vi "Add(U8).vi"(1 "Enable(T)":bool=TRUE, 2 "In":u8, 4 "n":u8=1) -> (6 "Out":u8=1)   [LabVIEW 2013]
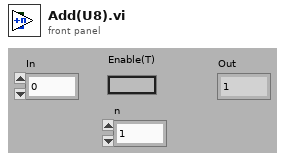
[diagram p1: front panel]
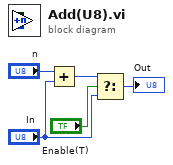
[diagram p0: block diagram]
diagram:
  n1 = Add(x="n", y="In") -> (x+y=w1:u8)
  n2 = Select(t=w1, s="Enable(T)", f="In") -> (s? t:f=→"Out":u8)
